vi "Username and Password.vi"() -> (2 "Logged In?":bool, 3 "User name out":string)   [LabVIEW 2023]
doc: "Simulates a user/password login prompt."
panel:
  in  "Cancel":bool
  in  "Password":string
  in  "User name":string
  in  "OK":bool
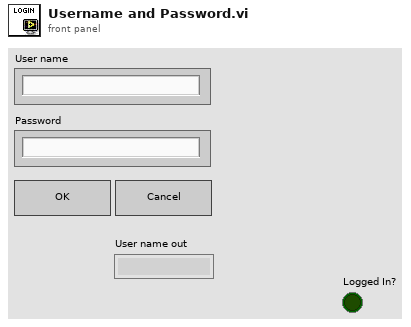
[diagram p1: front panel]
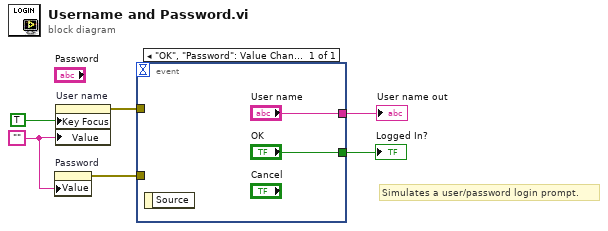
[diagram p0: block diagram]
diagram:
  w6 = ""
  # "Simulates a user/password login prompt."
  n1 = property on="Password" class="Str"("Value"=w6) -> (error out=w1:errorcluster)  [unwired: 2 in, 1 out]
  n2 = property on="User name" class="Str"("Key Focus"=TRUE, "Value"=w6) -> (error out=w2:errorcluster)  [unwired: 2 in, 1 out]
  n3 = event shown="[0] \"OK\", \"Password\": Value Change" {
    selector: _ -> [_]
    dyn-events: _ -> [_]
    timeout: _ -> [_]
    tunnel: ["OK"] -> w4
    tunnel: ["User name"] -> w3
    tunnel: w2 -> [_]
    tunnel: w1 -> [_]
    event "OK", "Password": Value Change {
      n4 = event-data() -> ()  [unwired: 1 in, 1 out]
    }
  }
  "Logged In?" <- w4
  "User name out" <- w3
